vi "Get Installed Software.vi"   [LabVIEW 2012, in "nisyscfg.lvlib"]
doc: "Retrieves the software installed on a system."
uses:
  <vilib>/nisyscfg/nisyscfg.lvlib
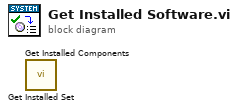
[diagram p0: block diagram]
diagram:
  n1 = call <vilib>:"Get Installed Set.vi"() -> ()  [unwired: 9 in, 3 out]
  n2 = call <vilib>:"Get Installed Components.vi"() -> ()  [unwired: 9 in, 3 out]
